vi "sv_Check for Array Change (spectrum).vi"(8 "error in (no error)":errorcluster, 11 "power spectrum":cluster{"f0":dbl, "df":dbl, "Spectrum":dbl[]} {"Spectrum" format="%.2f"; "df" format="%.2f"; "f0" format="%.2f"}) -> (0 "error out":errorcluster, 1 "Boolean":bool, 3 "dup power spectrum":cluster{"f0":dbl, "df":dbl, "Spectrum":dbl[]} {"Spectrum" format="%.2f"; "df" format="%.2f"; "f0" format="%.2f"})   [LabVIEW 2017]
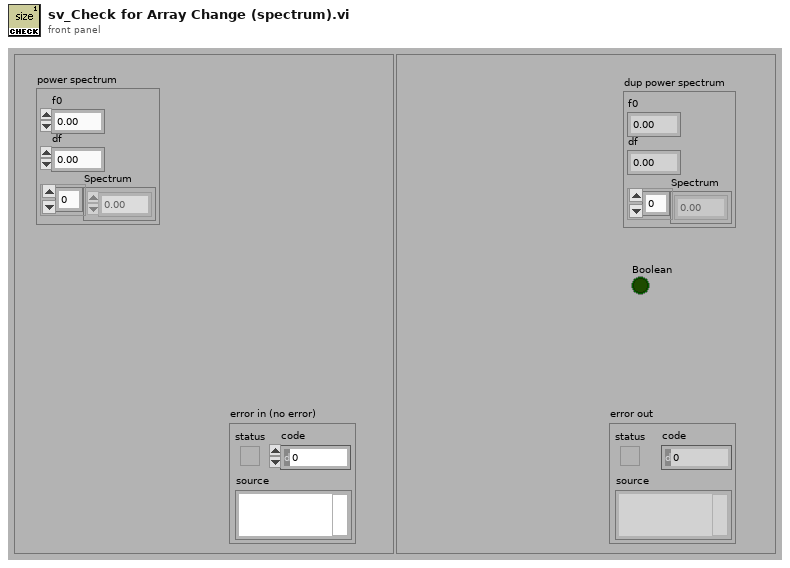
[diagram p1: front panel]
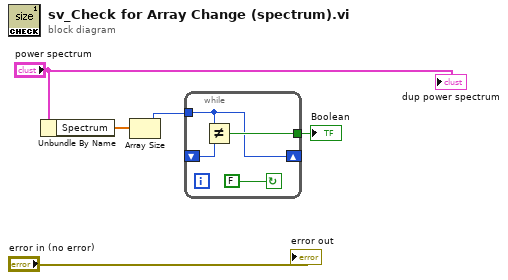
[diagram p0: block diagram]
diagram:
  n1 = Unbundle By Name("power spectrum") -> ("Spectrum"=w5:dbl[])
  n2 = Array Size(array=w5) -> (size(s)=w4:i32)
  n3 = while {
    tunnel: [w8] -> w3
    tunnel: w4 -> [w6]
    shift-left: _ -> [w7]
    shift-right: [w6] -> _
    stop <- FALSE continue-if-true
    n4 = Not Equal?(x=w6, y=w7) -> (x != y?=w8:bool)
  }
  "Boolean" <- w3
  "error out" <- "error in (no error)"
  "dup power spectrum" <- "power spectrum"
